vi "Test Launch Single Runner with Test Case.vi"(8 "error in (no error)":errorcluster, 11 "Test Runner Test in":refnum<class "Test Runner Test.lvclass">) -> (0 "error out":errorcluster, 3 "Test Runner Test out":refnum<class "Test Runner Test.lvclass">)   [LabVIEW 2020, in "Test Runner Test.lvclass"]
uses:
  Test Runner Test.lvclass
  C:/git/astemes-lunit/source/Framework/Result Observer/Result Observer.lvclass
  source/Core/LUnit Test Suite/LUnit Test Suite.lvclass
  C:/git/astemes-lunit/source/Core/Runnable/Runnable.lvclass
  source/Framework/Single Thread Test Runner/Single Thread Test Runner.lvclass
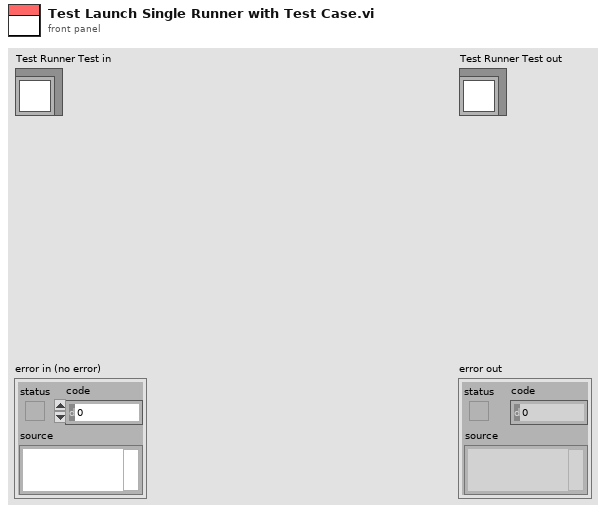
[diagram p1: front panel]
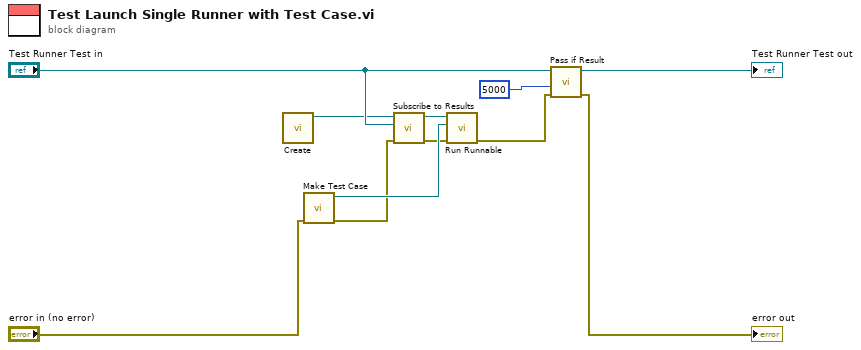
[diagram p0: block diagram]
diagram:
  n1 = call "Create.vi"() -> ("Single Thread Test Runner out"=w1:refnum<class "Single Thread Test Runner.lvclass">)  [unwired: 10 in, 1 out]
  n2 = call "Make Test Case.vi"("error in (no error)"="error in (no error)") -> ("error out"=w3:errorcluster, "LUnit Test Suite V2 out"=w11:refnum<class "LUnit Test Suite.lvclass">)  [unwired: 9 in]
  n3 = call-dynamic "Subscribe to Results.vi"("error in (no error)"=w3, "Result Observer"="Test Runner Test in", "Single Thread Test Runner In"=w1) -> ("error out"=w2:errorcluster, "Single Thread Test Runner Out"=w5:refnum<class "Single Thread Test Runner.lvclass">)  [unwired: 7 in]
  n4 = call-dynamic "Run Runnable.vi"("error in (no error)"=w2, "Runnable"=w11, "Single Thread Test Runner In"=w5) -> ("error out"=w9:errorcluster)  [unwired: 7 in, 1 out]
  n5 = call "Pass if Result.vi"("error in (no error)"=w9, "timeout in ms (0)"=5000, "Test Runner Test in"="Test Runner Test in") -> ("error out"=→"error out":errorcluster, "Test Runner Test out"=→"Test Runner Test out":refnum<class "Test Runner Test.lvclass">)  [unwired: 7 in]
